vi "Async Frametag.vi"(6 "Last Grab":bool, 7 "Arm Async Frametag":bool, 9 "Period Clock received":bool, 10 "Stop Trigger received":bool, 11 "Advance Trigger received":bool) -> (1 "End of Acquisition":bool, 2 "End of Grab":bool, 3 "Send Async Frametag":bool, 5 "Arm Async Frametag Out":bool)   [LabVIEW 2014]
panel:
  # "Copyright 2014 Vidrio Technologies\nScanImage 5 software is licensed under the Apache License, Version 2.0 (the \"License\"); you may not use any files contained\nwithin the ScanImage 5 release except in compliance with the License. You may obtain a copy of the License at\n http://www.apache.org/licenses/LICENSE-2.0\nUnless required by applicable law or agreed to in writing, software distributed under the License is distributed on an\n\"AS IS\" BASIS, WITHOUT WARRANTIES OR CONDITIONS OF ANY KIND, either express or implied. See the License for the\n specific language governing permissions and limitations under the License."
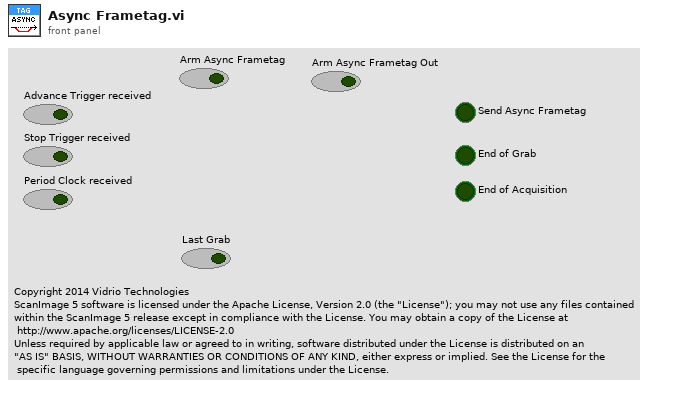
[diagram p1: front panel]
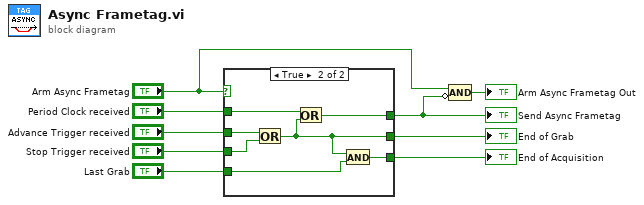
[diagram p0: block diagram]
diagram:
  n1 = case shown="True" "Arm Async Frametag" {
    tunnel: "Stop Trigger received" -> [_ w16]
    tunnel: [_ w15] -> w9
    tunnel: "Advance Trigger received" -> [_ w14]
    tunnel: [_ w13] -> w1
    tunnel: [_ w12] -> w8
    tunnel: "Period Clock received" -> [_ w11]
    tunnel: "Last Grab" -> [_ w10]
    frame False {
    }
    frame True {
      n2 = Or(x=w14, y=w16) -> (x .or. y?=w12:bool)
      n3 = Or(x=w11, y=w12) -> (x .or. y?=w13:bool)
      n4 = And(x=w12, y=w10) -> (x .and. y?=w15:bool)
    }
  }
  "End of Acquisition" <- w9
  "End of Grab" <- w8
  "Send Async Frametag" <- w1
  n5 = Compound Arithmetic op=AND("Arm Async Frametag", invert w1) -> (→"Arm Async Frametag Out":bool)
